vi "log2server.vi"(4 "error in":errorcluster) -> (0 "error out":errorcluster, 2 "msgs":string[](array[string]), 3 "cluster":T1)   [LabVIEW 2010]
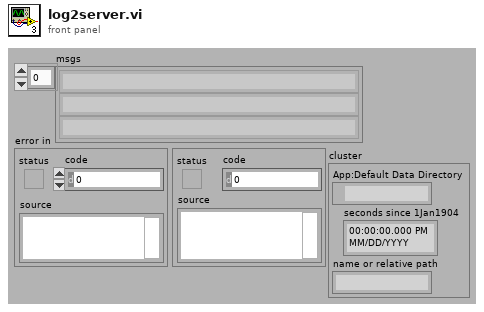
[diagram p1: front panel]
types:
  T1 = cluster{"App:Default Data Directory":path, "seconds since 1Jan1904":timestamp, "name or relative path":string}
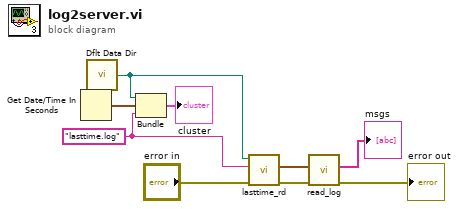
[diagram p0: block diagram]
diagram:
  w2 = "lasttime.log" ("name or relative path")
  n1 = Get Date/Time In Seconds() -> (seconds since 1Jan1904=w4:timestamp)
  n2 = call <vilib>:"Dflt Data Dir.vi"() -> ("App:Default Data Directory"=w3:path)
  n3 = Bundle("App:Default Data Directory"=w3, "seconds since 1Jan1904"=w4, "name or relative path"=w2) -> (→"cluster":T1)  [unwired: 1 in]
  n4 = call "lasttime_rd.vi"("error in"="error in", "name or relative path"=w2, "base path"=w3) -> ("error out"=w7:errorcluster, "time stamp"=w8:timestamp)  [unwired: 2 in, 1 out]
  n5 = call "read_log.vi"("error in"=w7, "last_time"=w8) -> ("error out"=→"error out":errorcluster, "msgs"=→"msgs":string[])  [unwired: 4 in]
